vi "finalize.vi"(8 "error in (no error)":errorcluster, 11 "object in":refnum<class "SQLiteConnection.lvclass">) -> (0 "error out":errorcluster, 3 "object out":refnum<class "SQLiteConnection.lvclass">)   [LabVIEW 2019, in "SQLiteConnection.lvclass"]
uses:
  SQLiteConnection.lvclass
  SQLiteConnection.lvclass/SQLiteConnection.ctl
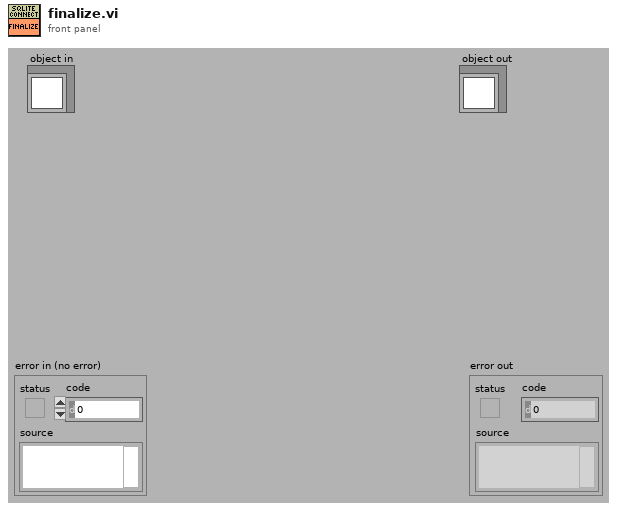
[diagram p1: front panel]
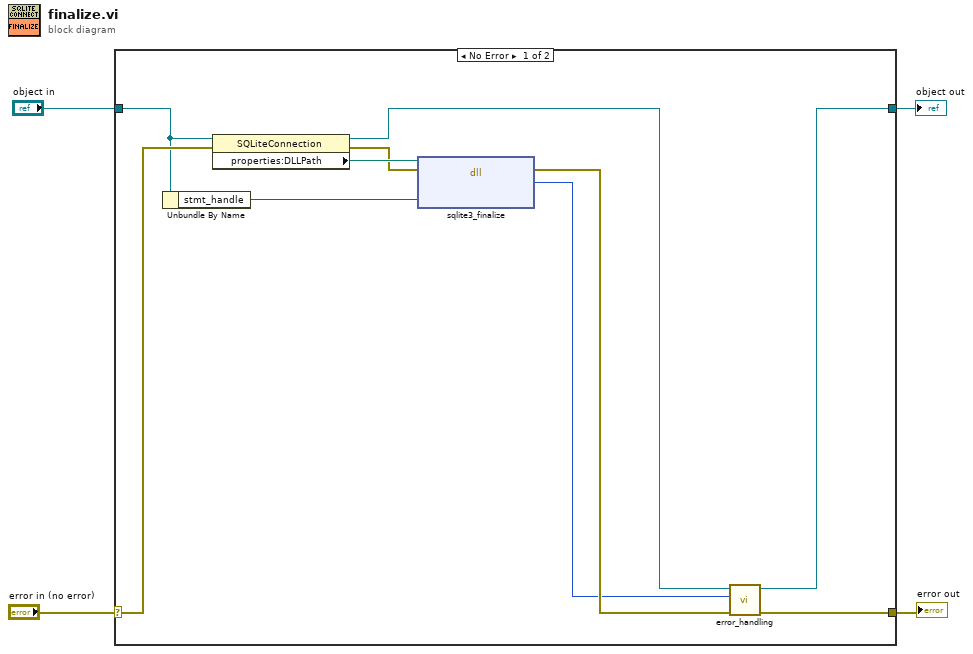
[diagram p0: block diagram]
diagram:
  n1 = case shown="No Error" "error in (no error)" {
    selector: "error in (no error)" -> [w9 w16]
    tunnel: [w13 w16] -> w3
    tunnel: [w10 w15] -> w1
    tunnel: "object in" -> [w7 w15]
    frame No Error {
      n2 = Unbundle By Name(w7) -> ("stmt_handle"=w12:u64)
      n3 = property class="SQLiteConnection"(reference=w7, error in=w9) -> (reference out=w6:refnum<class "SQLiteConnection.lvclass">, error out=w5:errorcluster, "properties:DLLPath"=w8:path)
      n4 = dll-call lib="D:/Users/mcarl/Documents/LabVIEW Projects/OW-PIKO/OW-PIKO Software/sqlite3.dll" fn="sqlite3_finalize"(path in=w8, error in=w5, "stmt_pointer"=w12) -> (error out=w14:errorcluster, "return type"=w11:i32)  [unwired: 2 in, 1 out]
      n5 = call "error_handling.vi"("error in (no error)"=w14, "error handle"=w11, "object in"=w6) -> ("error out"=w13:errorcluster, "object out"=w10:refnum<class "SQLiteConnection.lvclass">)  [unwired: 7 in]
    }
    frame Error {
    }
  }
  "error out" <- w3
  "object out" <- w1
